vi "MPPT.vi"() -> ()   [LabVIEW 2018]
uses:
  <vilib>/MakerHub/LINX/Public/Peripherals/Digital/Digital Write 1 Chan.vi
  <vilib>/MakerHub/LINX/Public/Peripherals/PWM/PWM Set Duty Cycle 1 Chan.vi
  <vilib>/MakerHub/LINX/Public/Peripherals/Analog/Analog Read 1 Chan.vi
  <vilib>/MakerHub/LINX/Public/Peripherals/Digital/Digital Write N Chans.vi
  <vilib>/MakerHub/LINX/Public/Peripherals/Analog/Analog Read N Chans.vi
  <vilib>/MakerHub/LINX/Private/Local IO/LinxDigitalWrite.vi
  <vilib>/MakerHub/LINX/Public/Utilities/Check Channel.vi
  <vilib>/MakerHub/LINX/Private/Local IO/LinxAnalogRead.vi
  <vilib>/MakerHub/LINX/Public/Utilities/Open Serial.vi
  <vilib>/MakerHub/LINX/Private/Utilties/Generate Error.vi
  <vilib>/MakerHub/LINX/Public/Peripherals/PWM/PWM Set Duty Cycle N Chans.vi
  <vilib>/MakerHub/LINX/LMH-LINX.lvlib
panel:
  in  "Röle-1":bool
  in  "Röle-2":bool
  in  "Koruma":bool
  in  "CV/CC":bool
  in  "MPPT":bool
  out "V":string[][](table)
  in  "V":dbl[](array[numeric])
  out "I-V Curve":cluster{"Y":dbl[], "Y":dbl[]}[](graph)
  in  "V":dbl[](array[numeric])
  in  "P":dbl[](array[numeric])
  in  "I":dbl[](array[numeric])
  out "OutputPowerDelta":dbl(graph)
  out "Potentioal Value":dbl(graph)
  out "Target Output Voltage":dbl(graph)
  in  "Duty Cycle (0-1)":dbl
  in  "stop":bool
  out "P in":dbl(graph)
  out "I out":dbl(graph)
  out "P out":dbl(graph)
  out "V out":dbl(graph)
  out "I in":dbl(graph)
  out "V in":dbl(graph)
  in  "Baud Rate":u32
  in  "Serial Port":refnum<visa-resource-name>="N/A"
  # "MAKSİMUM GÜÇ NOKTASI İZLEYİCLİ FOTOVOLTAİK\nSYSTEMİN LABVİEW TABANLI KONTROLÜ İZLEMESİ\n\n                  Doç.Dr. Ahmet AFŞİN KULAKSIZ\n                          Abdulkadir MÜHENDİS\n                                  KONYA - 2020"
  # "Recorded Arrayes Lists"
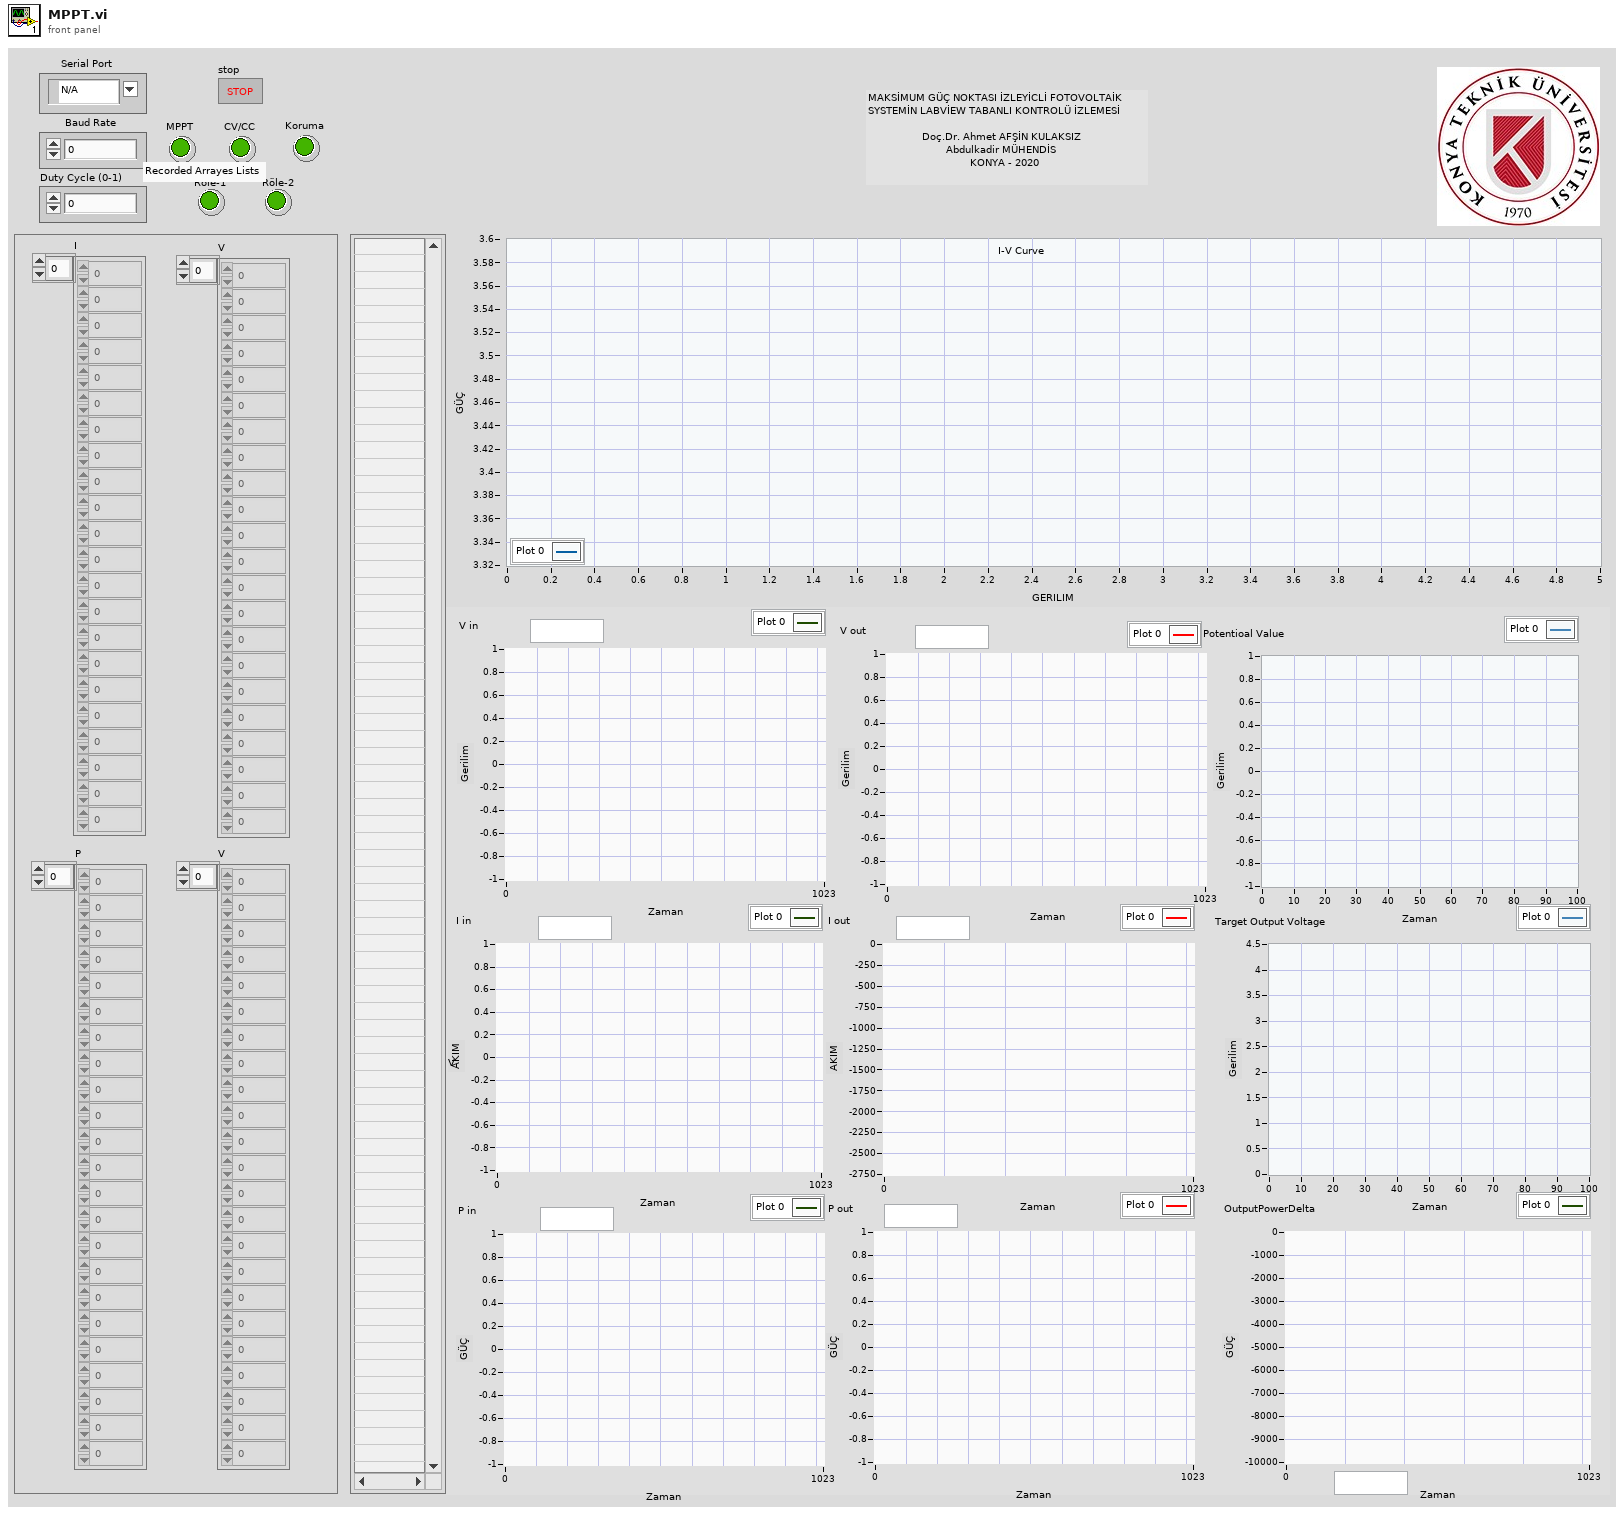
[diagram p1: front panel]
types:
  T1 = typedef "LMH-LINX.lvlib/LINX Ref.ctl" = cluster{"IO":T2, "Interface":T3, "LINX Device Config":T4}
  T2 = typedef "LMH-LINX.lvlib/Platform.ctl" = enum16{"Remote", "Local"}
  T3 = typedef "LMH-LINX.lvlib/Interface.ctl" = enum16{"Serial", "TCP"}
  T4 = typedef "LMH-LINX.lvlib/Device.lvlib/LINX Device Config.ctl" = cluster{"Interface":T3, "COM Port":refnum<visa-resource-name>, "TCP Configuration":T5, "Device Family":u8, "Device ID":u8, "Device Name":string, "TCP Ref":refnum<k5>, "Channels":T6}
  T5 = typedef "LMH-LINX.lvlib/Device.lvlib/TCP Config.ctl" = cluster{"IP Address":string, "Port":u16}
  T6 = typedef "LMH-LINX.lvlib/Channels.ctl" = cluster{"DI":u8[], "DO":u8[], "AI":u8[], "AO":u8[], "PWM":u8[], "QE":u8[], "UART":u8[], "I2C 2":u8[], "SPI":u8[], "CAN":u8[], "Servo":u8[], "AI Ref (V)":dbl, "AI Resolution (Bits)":u8, "AO Ref (V)":dbl, "AO Resolution (Bits)":u8}
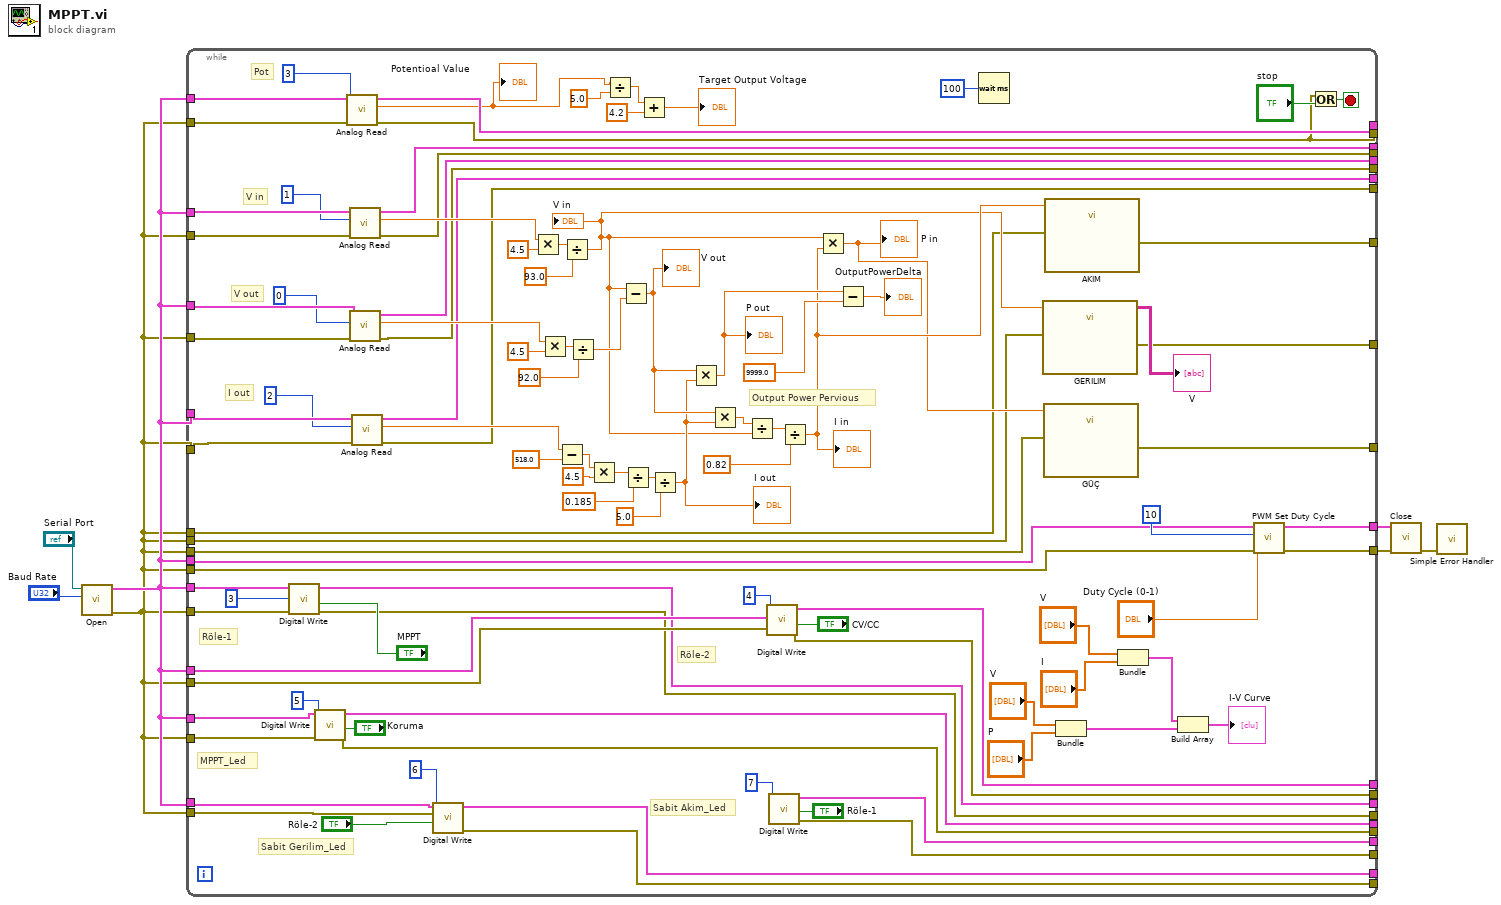
[diagram p0: block diagram]
diagram:
  n1 = call-poly <vilib>:"Open.vi"("Baud Rate Override"="Baud Rate", "Serial Port"="Serial Port") -> ("Error Out"=w3:errorcluster, "LINX Resource"=w4:T1)  [unwired: 7 in, 1 out]
  n2 = while {
    tunnel: [w85] -> _
    tunnel: [w34] -> _
    tunnel: [w84] -> _
    tunnel: [w83] -> _
    tunnel: [w82] -> _
    tunnel: [w81] -> _
    tunnel: [w80] -> _
    tunnel: [w79] -> _
    tunnel: w4 -> [w78]
    tunnel: w4 -> [w77]
    tunnel: w4 -> [w76]
    tunnel: w4 -> [w75]
    tunnel: w3 -> [w74]
    tunnel: w3 -> [w73]
    tunnel: w3 -> [w72]
    tunnel: w3 -> [w71]
    tunnel: [w42] -> _
    tunnel: [w41] -> _
    tunnel: [w40] -> _
    tunnel: w3 -> [w39]
    tunnel: w3 -> [w38]
    tunnel: w3 -> [w37]
    tunnel: w3 -> [w36]
    tunnel: w4 -> [w35]
    tunnel: w4 -> [w33]
    tunnel: w4 -> [w32]
    tunnel: w4 -> [w31]
    tunnel: w4 -> [w30]
    tunnel: w3 -> [w29]
    tunnel: w3 -> [w28]
    tunnel: w3 -> [w27]
    tunnel: w3 -> [w26]
    tunnel: [w20] -> _
    tunnel: [w19] -> w2
    tunnel: [w18] -> w1
    tunnel: [w17] -> _
    tunnel: [w16] -> _
    tunnel: [w15] -> _
    tunnel: [w14] -> _
    tunnel: [w13] -> _
    tunnel: [w12] -> _
    tunnel: [w11] -> _
    tunnel: [w10] -> _
    tunnel: [w9] -> _
    stop <- w88 stop-if-true
    # "Output Power Pervious"
    # "Sabit Akim_Led"
    # "Sabit Gerilim_Led"
    # "MPPT_Led"
    # "Röle-2"
    # "Röle-1"
    # "Pot"
    # "V in"
    # "V out"
    # "I out"
    n3 = call-poly <vilib>:"Digital Write.vi"("Error In"=w29, "Output Value"="MPPT", "DO Channel"=u8 3, "LINX Resource"=w33) -> ("Error Out"=w15:errorcluster, "LINX Resource"=w16:T1)  [unwired: 6 in]
    n4 = call-poly <vilib>:"Digital Write.vi"("Error In"=w27, "Output Value"="Koruma", "DO Channel"=u8 5, "LINX Resource"=w31) -> ("Error Out"=w13:errorcluster, "LINX Resource"=w14:T1)  [unwired: 6 in]
    n5 = call-poly <vilib>:"Analog Read.vi"("Error In"=w74, "Analog Channel"=u8 3, "LINX Resource"=w78) -> ("Error Out"=w34:errorcluster, "Voltage"=w8:dbl, "LINX Resource"=w85:T1)  [unwired: 5 in, 1 out]
    "Potentioal Value" <- w8
    n6 = call-poly <vilib>:"Analog Read.vi"("Error In"=w73, "Analog Channel"=u8 1, "LINX Resource"=w77) -> ("Error Out"=w83:errorcluster, "Voltage"=w99:dbl, "LINX Resource"=w84:T1)  [unwired: 5 in, 1 out]
    n7 = call-poly <vilib>:"Analog Read.vi"("Error In"=w72, "Analog Channel"=u8 0, "LINX Resource"=w76) -> ("Error Out"=w81:errorcluster, "Voltage"=w93:dbl, "LINX Resource"=w82:T1)  [unwired: 5 in, 1 out]
    n8 = call-poly <vilib>:"Analog Read.vi"("Error In"=w71, "Analog Channel"=u8 2, "LINX Resource"=w75) -> ("Error Out"=w79:errorcluster, "Voltage"=w86:dbl, "LINX Resource"=w80:T1)  [unwired: 5 in, 1 out]
    n9 = call-poly <vilib>:"Digital Write.vi"("Error In"=w26, "Output Value"="Röle-2", "DO Channel"=u8 6, "LINX Resource"=w30) -> ("Error Out"=w11:errorcluster, "LINX Resource"=w12:T1)  [unwired: 6 in]
    n10 = Multiply(x=w99, y=4.5) -> (x*y=w98:dbl)
    n11 = Multiply(x=w93, y=4.5) -> (x*y=w95:dbl)
    n12 = Subtract(x=w86, y=518.0) -> (x-y=w106:dbl)
    n13 = Divide(x=w98, y=93.0) -> (x/y=w44:dbl)
    "V in" <- w44
    n14 = Divide(x=w95, y=92.0) -> (x/y=w92:dbl)
    n15 = Multiply(x=w106, y=4.5) -> (x*y=w104:dbl)
    n16 = Divide(x=w8, y=5.0) -> (x/y=w108:dbl)
    n17 = Subtract(x=w44, y=w92) -> (x-y=w69:dbl)
    "V out" <- w69
    n18 = Divide(x=w104, y=0.185) -> (x/y=w102:dbl)
    n19 = Add(x=w108, y=4.2) -> (x+y=→"Target Output Voltage":dbl)
    n20 = Divide(x=w102, y=5.0) -> (x/y=w68:dbl)
    "I out" <- w68
    n21 = Multiply(x=w69, y=w68) -> (x*y=w56:dbl)
    "P out" <- w56
    n22 = Multiply(x=w69, y=w68) -> (x*y=w91:dbl)
    n23 = Divide(x=w91, y=w44) -> (x/y=w90:dbl)
    n24 = call-poly <vilib>:"Digital Write.vi"("Error In"=w28, "Output Value"="CV/CC", "DO Channel"=u8 4, "LINX Resource"=w32) -> ("Error Out"=w17:errorcluster, "LINX Resource"=w20:T1)  [unwired: 6 in]
    n25 = call-poly <vilib>:"Digital Write.vi"("Output Value"="Röle-1", "DO Channel"=u8 7) -> ("Error Out"=w9:errorcluster, "LINX Resource"=w10:T1)  [unwired: 8 in]
    n26 = Divide(x=w90, y=0.82) -> (x/y=w45:dbl)
    "I in" <- w45
    n27 = Multiply(x=w44, y=w45) -> (x*y=w43:dbl)
    "P in" <- w43
    n28 = Subtract(x=w56, y=9999.0) -> (x-y=→"OutputPowerDelta":dbl)
    n29 = Wait (ms)(milliseconds to wait=u32 100) -> ()  [unwired: 1 out]
    n30 = call "GERILIM"("error in (no error)"=w38, "Signals"=w44) -> ("error out"=w41:errorcluster, "Table"=→"V":string[][])  [unwired: 3 in, 5 out]
    n31 = call "GÜÇ"("error in (no error)"=w37, "Signals"=w43) -> ("error out"=w40:errorcluster)  [unwired: 3 in, 6 out]
    n32 = call "AKIM"("error in (no error)"=w39, "Signals"=w45) -> ("error out"=w42:errorcluster)  [unwired: 3 in, 6 out]
    n33 = Bundle("V"="V", "P"="P") -> (w49:cluster{"V":dbl[], "P":dbl[]})  [unwired: 1 in]
    n34 = Bundle("V"="V", "I"="I") -> (w50:cluster{"V":dbl[], "I":dbl[]})  [unwired: 1 in]
    n35 = Build Array(w50, w49) -> (→"I-V Curve":cluster{"V":dbl[], "P":dbl[]}[])
    n36 = call-poly <vilib>:"PWM Set Duty Cycle.vi"("Error In"=w36, "Duty Cycle (0-1)"="Duty Cycle (0-1)", "PWM Channel"=u8 10, "LINX Resource"=w35) -> ("Error Out"=w18:errorcluster, "LINX Resource"=w19:T1)  [unwired: 6 in]
    n37 = Or(x=w34, y="stop") -> (x .or. y?=w88:bool)
  }
  n38 = call <vilib>:"Close.vi"("Error In"=w1, "LINX Resource"=w2) -> ("Error Out"=w5:errorcluster)  [unwired: 9 in]
  n39 = call <vilib>:"Simple Error Handler.vi"("error in (no error)"=w5) -> ()  [unwired: 4 in, 5 out]
